vi "delete tag.vi"(7 "owner ID":string, 8 "error in":errorcluster, 10 "tag name":string, 11 "engine configuration in":refnum<class "engine configuration.lvclass">) -> (0 "error out":errorcluster, 3 "engine configuration out":refnum<class "engine configuration.lvclass">)   [LabVIEW 2013, in "engine configuration.lvclass"]
uses:
  engine configuration.lvclass
  <vilib>/NI/Tag Bus/tag/tag descriptor.lvclass
  <vilib>/NI/Tag Bus/tag/tag descriptor.lvclass/tag descriptor.ctl
  engine configuration.lvclass/engine configuration.ctl
  <vilib>/NI/Tag Bus/tag/write tag name.vi
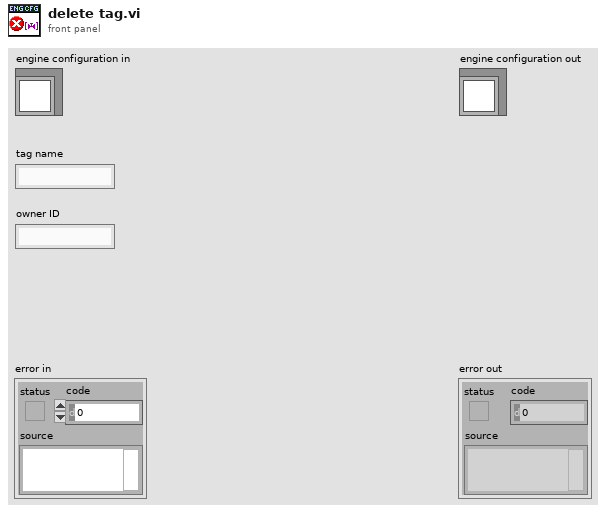
[diagram p1: front panel]
types:
  T1 = typedef "engine configuration.lvclass/Tag Info.ctl" = cluster{"Tag":refnum<class "tag descriptor.lvclass">, "Writer":string, "Readers":string[], "Owning ID":string}
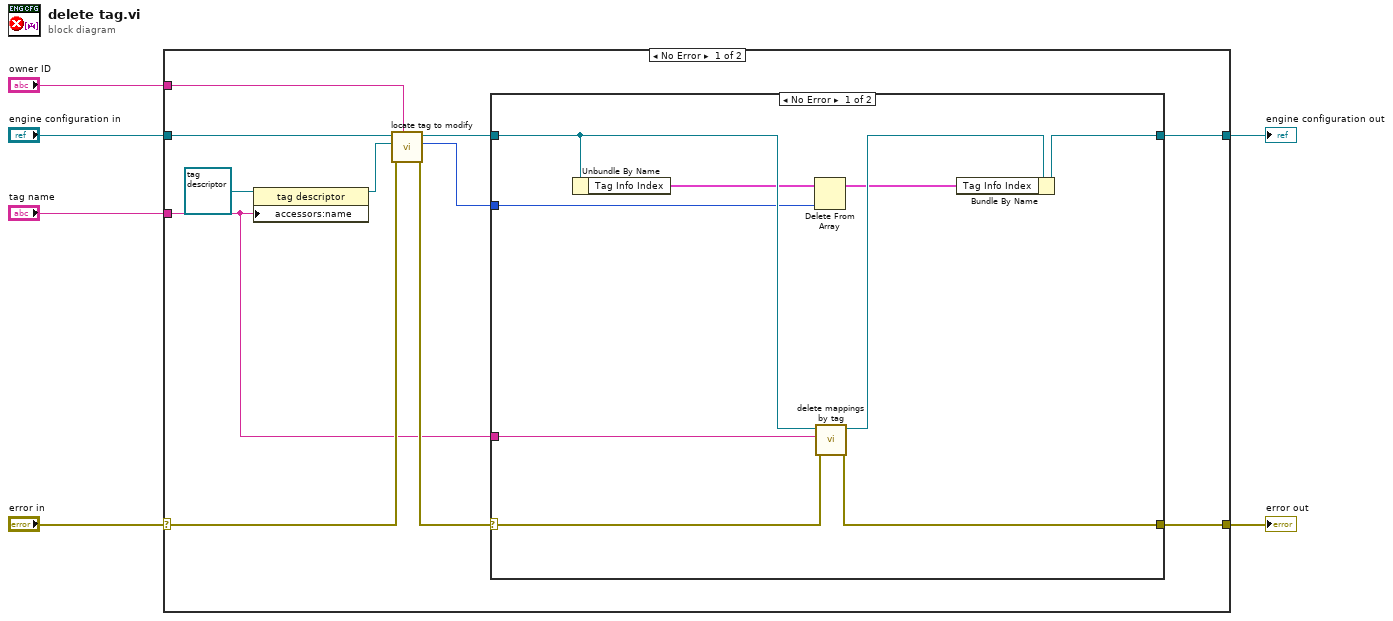
[diagram p0: block diagram]
diagram:
  n1 = case shown="No Error" "error in" {
    selector: "error in" -> [w11 w30]
    tunnel: [w16 w30] -> w2
    tunnel: [w17 w29] -> w3
    tunnel: "engine configuration in" -> [w15 w29]
    tunnel: "tag name" -> [w7 _]
    tunnel: "owner ID" -> [w14 _]
    frame No Error {
      n2 = property class="tag descriptor"(reference=refnum<class "tag descriptor.lvclass"> refnum ("tag descriptor"), "accessors:name"=w7) -> (reference out=w12:refnum<class "tag descriptor.lvclass">)  [unwired: 1 in, 1 out]
      n3 = call "locate tag to modify.vi"("owner ID"=w14, "error in"=w11, "tag descriptor"=w12, "engine configuration in"=w15) -> ("error out"=w9:errorcluster, "index"=w8:i32, "engine configuration out"=w10:refnum<class "engine configuration.lvclass">)  [unwired: 5 in]
      n4 = case shown="No Error" w9 {
        selector: w9 -> [w20 w27]
        tunnel: w10 -> [w25 w28]
        tunnel: [w26 w28] -> w17
        tunnel: [w24 w27] -> w16
        tunnel: w8 -> [w21 _]
        tunnel: w7 -> [w18 _]
        frame No Error {
          n5 = Unbundle By Name(w25) -> ("Tag Info Index"=w22:T1[])
          n6 = Delete From Array(array=w22, index=w21) -> (array with subset deleted=w19:T1[])  [unwired: 1 in, 1 out]
          n7 = call "delete mappings by tag.vi"("error in"=w20, "tag name"=w18, "engine configuration in"=w25) -> ("error out"=w24:errorcluster, "engine configuration out"=w23:refnum<class "engine configuration.lvclass">)  [unwired: 7 in]
          n8 = Bundle By Name(cluster=w23, "Tag Info Index"=w19) -> (w26:refnum<class "engine configuration.lvclass">)
        }
        frame Error {
        }
      }
    }
    frame Error {
    }
  }
  "error out" <- w2
  "engine configuration out" <- w3
